vi "NewConnection.vi"(8 "error in (no error)":errorcluster, 10 "Connection Information":T1, 11 "TCP_Server in":refnum<class "TCP_Server.lvclass">) -> (0 "error out":errorcluster, 3 "TCP_Server out":refnum<class "TCP_Server.lvclass">)   [LabVIEW 2023, in "TCP_Server.lvlib" / "TCP_Server.lvclass"]
uses:
  TCP_Server.lvclass
  C:/Program Files (x86)/National Instruments/LabVIEW 2023/vi.lib/ActorFramework/Actor/Actor.lvclass
  TCP_Listener/TypeDefinitions/ConnectionInformation.ctl
  TCP_Server.lvclass/TCP_Server.ctl
  TypeDeclarations/ServerConnection.ctl
  <vilib>/ActorFramework/Message Enqueuer/Message Enqueuer.lvclass
  <vilib>/ActorFramework/Message Enqueuer/Message Priority.ctl
  <vilib>/ActorFramework/Actor/Actor.lvclass/Actor.ctl
  <vilib>/ActorFramework/Message Enqueuer/Message Enqueuer.lvclass/Message Enqueuer.ctl
  TCP_Server Messages/AddConnection Msg/AddConnection Msg.lvclass/AddConnection Msg.ctl
  TCP_Server_Connection_Handler/TCP_Server_Connection_Handler/TCP_Server_Connection_Handler.lvclass
  TCP_Server_Connection_Handler/TCP_Server_Connection_Handler Messages/Write Connection Information Msg/Write Connection Information Msg.lvclass/Write Connection Information Msg.ctl
  TCP_Server_Connection_Handler/TCP_Server_Connection_Handler Messages/SendString Msg/SendString Msg.lvclass/SendString Msg.ctl
  <vilib>/ActorFramework/Message Enqueuer/Init from Existing Queue.vi
  <vilib>/ActorFramework/Message Enqueuer/Enqueue.vi
  TCP_Server Messages/AddConnection Msg/AddConnection Msg.lvclass
  C:/Program Files (x86)/National Instruments/LabVIEW 2023/vi.lib/ActorFramework/Message/Message.lvclass
  TCP_Server_Connection_Handler/TCP_Server_Connection_Handler Messages/Write Connection Information Msg/Write Connection Information Msg.lvclass
  TCP_Server_Connection_Handler/TCP_Server_Connection_Handler Messages/SendString Msg/SendString Msg.lvclass
  <vilib>/ActorFramework/Stop Msg/Stop Msg.lvclass
  <vilib>/ActorFramework/Message Priority Queue/Priority Enqueue.vi
  <vilib>/ActorFramework/Actor/Actor.lvclass
  TCP_Listener/TCP_Listener.lvlib
  TCP_Server.lvlib
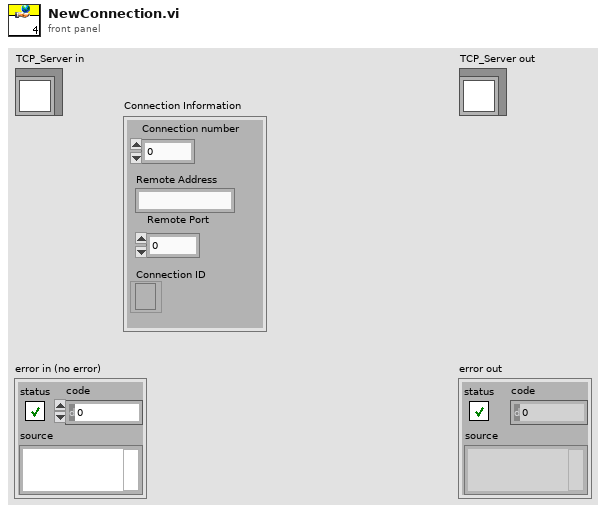
[diagram p1: front panel]
types:
  T1 = typedef "TCP_Listener.lvlib/ConnectionInformation.ctl" = cluster{"Connection number":i32, "Remote Address":string, "Remote Port":u16, "Connection ID":refnum<k5>}
  T2 = typedef "Actor Framework.lvlib/Message Enqueuer.lvclass/Message Priority.ctl" = enum16{"Low", "Normal", "High"}
  T3 = typedef "TCP_Server.lvlib/ServerConnection.ctl" = cluster{"Connection Handlers's Enqueuer":refnum<class "Message Enqueuer.lvclass">, "Connection Window's Enqueuer":refnum<class "Message Enqueuer.lvclass">, "Connection Information":T1}
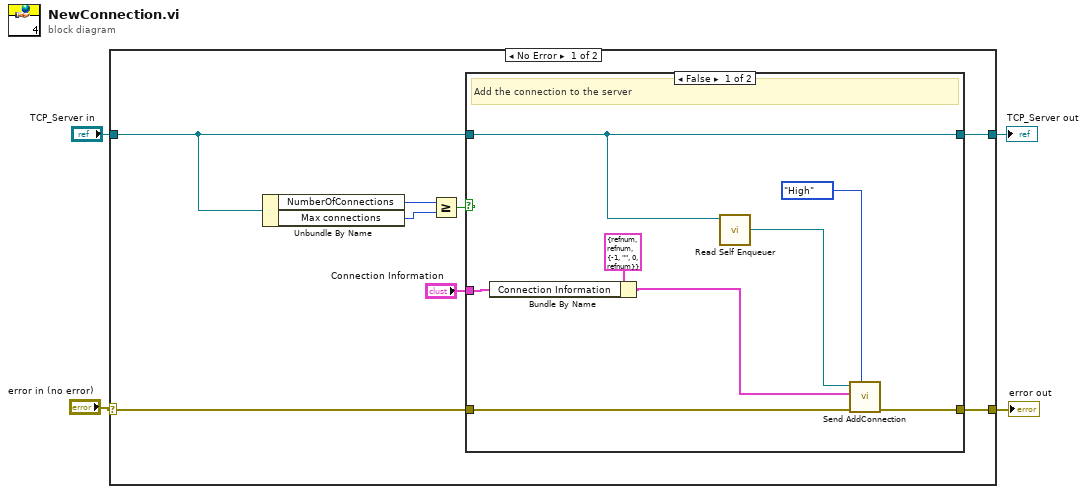
[diagram p0: block diagram]
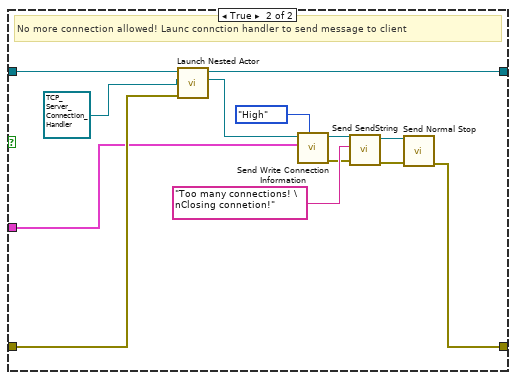
[diagram p2: hidden frame]
diagram:
  n1 = case shown="No Error" "error in (no error)" {
    selector: "error in (no error)" -> [w8 w35]
    tunnel: [w7 w35] -> w3
    tunnel: [w9 w34] -> w2
    tunnel: "TCP_Server in" -> [w10 w34]
    frame No Error {
      n2 = Unbundle By Name(w10) -> ("NumberOfConnections"=w6:i32, "Max connections"=w5:i32)
      n3 = Greater Or Equal?(x=w6, y=w5) -> (x >= y?=w12:bool)
      n4 = case shown="False" w12 {
        tunnel: "Connection Information" -> [w13 w29]
        tunnel: w10 -> [w17 w33]
        tunnel: [w17 w32] -> w9
        tunnel: w8 -> [w20 w31]
        tunnel: [w19 w25] -> w7
        frame False {
          # "Add the connection to the server"
          n5 = Bundle By Name(cluster=T3 {"Connection Handlers's Enqueuer"=refnum, "Connection Window's Enqueuer"=refnum, "Connection Information"={"Connection number"=-1, "Remote Address"="", "Remote Port"=0, "Connection ID"=refnum}} ("Connection"), "Connection Information"=w13) -> (w14:T3)
          n6 = call <vilib>:"Read Self Enqueuer.vi"("Actor"=w17) -> ("Self Enqueuer"=w18:refnum<class "Message Enqueuer.lvclass">)  [unwired: 10 in]
          n7 = call "Send AddConnection.vi"("Message Priority (Normal)"=Message_Priority."High", "error in (no error)"=w20, "Connection"=w14, "Message Enqueuer"=w18) -> ("error out"=w19:errorcluster)  [unwired: 6 in, 1 out]
        }
        frame True {
          # "No more connection allowed! Launc connction handler to send message to client"
          n8 = call <vilib>:"Launch Nested Actor.vi"("error in (no error)"=w31, "Nested Actor"=refnum<class "TCP_Server_Connection_Handler.lvclass"> refnum ("TCP_Server_Connection_Handler.lvlib:TCP_Server_Connection_Handler.lvclass"), "Caller Actor in"=w33) -> ("Nested Actor's Enqueuer"=w30:refnum<class "Message Enqueuer.lvclass">, "Caller Actor out"=w32:refnum<class "TCP_Server.lvclass">)  [unwired: 6 in, 1 out]
          n9 = call "Send Write Connection Information.vi"("Message Priority (Normal)"=Message_Priority."High", "Connection Information"=w29, "Message Enqueuer"=w30) -> ("error out"=w22:errorcluster, "Message Enqueuer out"=w23:refnum<class "Message Enqueuer.lvclass">)  [unwired: 7 in]
          n10 = call "Send SendString.vi"("error in (no error)"=w22, "Message"="Too many connections! \nClosing connetion!", "Message Enqueuer"=w23) -> ("error out"=w27:errorcluster, "Message Enqueuer out"=w26:refnum<class "Message Enqueuer.lvclass">)  [unwired: 7 in]
          n11 = call <vilib>:"Send Normal Stop.vi"("error in (no error)"=w27, "Message Enqueuer"=w26) -> ("error out"=w25:errorcluster)  [unwired: 9 in]
        }
      }
    }
    frame Error {
    }
  }
  "error out" <- w3
  "TCP_Server out" <- w2
